vi "AnalogInputVoltageSampleLoop.vi"   [LabVIEW 2018]
uses:
  AnalogInputSample.ctl
  <vilib>/rvi/Emulation/niFpgaGetClockAttributes.vi
  <vilib>/rvi/Emulation/niFpgaSctlEmulationGetInTimedLoop.vi
  <vilib>/rvi/Emulation/niFpgaEmulationReportErrorSimple.vi
  <vilib>/rvi/Emulation/niFpgaEmulationIsFPGAContextNoSignature.vi
  <vilib>/rvi/errors/niFpgaSetErrorForExecOnDevCompSimple.vi
  <vilib>/rvi/eio/common/nirviEmuReportErrorAndStop.vi
  <vilib>/rvi/DataTransferAndStorage/Container/Common/niFpgaContainerGetUniqueNameForEmu.vi
  <vilib>/rvi/FIFO/Fifo_Resource/nirvififoEmulationSetSize.vi
  <vilib>/rvi/FIFO/Fifo_Resource/nirviFifoEmulationQueueMgr.vi
  <instcachedir>/0/nirviFifoEmulationQueueMgr_E5CAEC123FF24DC58D834DCA3CDAA9B5.lvgen/nirviFifoEmulationQueueMgr_E5CAEC123FF24DC58D834DCA3CDAA9B5_002.vi
  <vilib>/Utility/error.llb/Clear Errors.vi
  <vilib>/rvi/FIFO/Fifo_Resource/nirvififoEmulationCreateLock.vi
  <vilib>/rvi/Emulation/niFpgaProcessEmulError.vi
  <vilib>/rvi/FIFO/Fifo_Resource/nirvififoEmulationObtainLock.vi
  <vilib>/rvi/FIFO/Fifo_Resource/nirvififoEmulationReleaseLock.vi
  <vilib>/rvi/occurrence/nirviWaitOnOccurrenceBase.vi
  <vilib>/rvi/errors/nirviReportUnexpectedCaseInternalError.vi
  <vilib>/rvi/errors/nirviReportUnexpectedCaseInternalError (U32).vi
  <vilib>/rvi/eio/common/nirviEmuTemplateMethod_errors.vi
  <vilib>/rvi/Memory/Memory_Emulation/niFpgaMemoryEmulationCacheClearOnFirstRun.vi
  <vilib>/rvi/Memory/Memory_Emulation/nirvimemoryEmulationManagerCache_MakeExclusive.vi
  <vilib>/rvi/Memory/Memory_Emulation/niFpgaMemoryEmulationValidateCache.vi
  <vilib>/rvi/Memory/Memory_Emulation/nirvimemoryEmulationManagerCache_InsertValue.vi
  <vilib>/rvi/Memory/Memory_Emulation/nirvimemoryEmulationManagerCache_ReleaseExclusive.vi
  <vilib>/rvi/Memory/Memory_Emulation/nirvimemoryEmulationManagerCache_GetValue.vi
  <vilib>/rvi/Memory/Memory_Emulation/nirvimemoryEmulationManagerCache_SetValue.vi
  <instcachedir>/0/nirviFifoEmulationQueueMgr_E5CAEC123FF24DC58D834DCA3CDAA9B5.lvgen/nirviFifoEmulationQueueMgr_E5CAEC123FF24DC58D834DCA3CDAA9B5_025.vi
  <vilib>/rvi/FIFO/Fifo_Resource/nirvififoEmulationDetermineInputValidOut.vi
  <vilib>/rvi/Emulation/niFpgaCriticalErrorInLSC.vi
  <vilib>/rvi/DataTransferAndStorage/Container/XNode/niFpgaContainer.xnode
  <vilib>/rvi/FIFO/Fifo_Resource/nirvififoEmulationRead.vi
  <vilib>/eio/EIONode/EIONode.xnode
  <vilib>/rvi/DataTransferAndStorage/Register/Emulation/niFpgaRegisterEmulation.vi
  <vilib>/rvi/FIFO/Fifo_Resource/nirvififoEmulationWrite.vi
types:
  T1 = typedef "AnalogInputSample.ctl" = cluster{"Sample":u64, "Timestamp":u64, "Raw1":sgl, "Raw2":sgl, "Raw3":sgl, "Raw4":sgl, "Raw5":sgl, "Raw6":sgl, "Raw7":sgl, "Raw8":sgl, "Raw9":sgl, "Raw10":sgl, "Raw11":sgl, "Raw12":sgl, "Raw13":sgl, "Raw14":sgl, "Raw15":sgl, "Raw16":sgl}
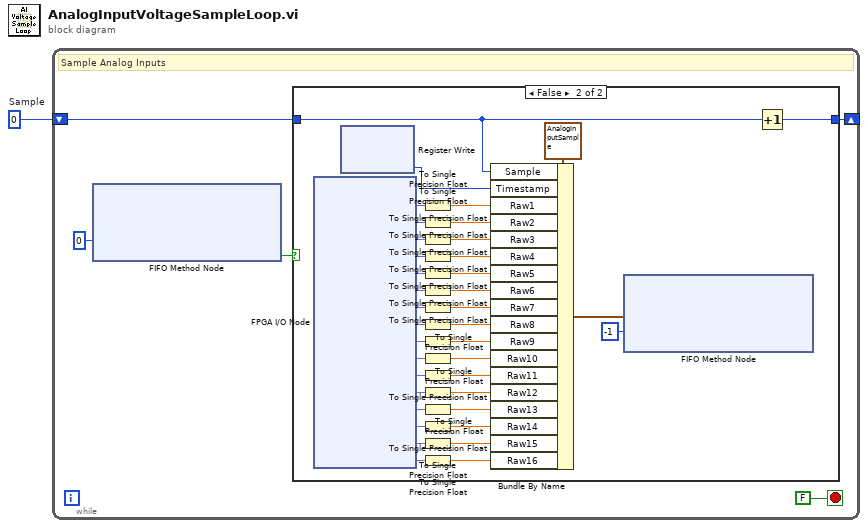
[diagram p0: block diagram]
diagram:
  w1 = u64 0  # Sample
  n1 = while {
    shift-right: [w2] -> _
    shift-left: w1 -> [w3]
    stop <- FALSE stop-if-true
    # "Sample Analog Inputs"
    n2 = xnode ("FIFO Method Node")("Timeout"=0) -> ("Timed Out?"=w5:bool)  [unwired: 1 in, 2 out]
    n3 = case shown="False" w5 {
      tunnel: w3 -> [w7 w27]
      tunnel: [w7 w26] -> w2
      frame True {
      }
      frame False {
        n4 = xnode "FPGA I/O Node"() -> ("Mod1/AI0"=w45:fxp<+/-,24,5>, "Mod1/AI1"=w44:fxp<+/-,24,5>, "Mod1/AI2"=w43:fxp<+/-,24,5>, "Mod1/AI3"=w42:fxp<+/-,24,5>, "Mod1/AI4"=w41:fxp<+/-,24,5>, "Mod1/AI5"=w40:fxp<+/-,24,5>, "Mod1/AI6"=w39:fxp<+/-,24,5>, "Mod1/AI7"=w38:fxp<+/-,24,5>, "Mod1/AI8"=w16:fxp<+/-,24,-4>, "Mod1/AI9"=w17:fxp<+/-,24,-4>, "Mod1/AI10"=w18:fxp<+/-,24,-4>, "Mod1/AI11"=w19:fxp<+/-,24,-4>, "Mod1/AI12"=w20:fxp<+/-,24,-4>, "Mod1/AI13"=w21:fxp<+/-,24,-4>, "Mod1/AI14"=w22:fxp<+/-,24,-4>, "Mod1/AI15"=w23:fxp<+/-,24,-4>)  [unwired: 16 in, 16 out]
        n5 = xnode "Register Write"() -> ("Data"=w25:u64)  [unwired: 1 in, 1 out]
        n6 = To Single Precision Float(number=w45) -> (single precision float=w37:sgl)
        n7 = To Single Precision Float(number=w44) -> (single precision float=w36:sgl)
        n8 = To Single Precision Float(number=w43) -> (single precision float=w35:sgl)
        n9 = To Single Precision Float(number=w42) -> (single precision float=w34:sgl)
        n10 = To Single Precision Float(number=w41) -> (single precision float=w33:sgl)
        n11 = To Single Precision Float(number=w40) -> (single precision float=w32:sgl)
        n12 = To Single Precision Float(number=w39) -> (single precision float=w31:sgl)
        n13 = To Single Precision Float(number=w38) -> (single precision float=w24:sgl)
        n14 = To Single Precision Float(number=w16) -> (single precision float=w15:sgl)
        n15 = To Single Precision Float(number=w17) -> (single precision float=w14:sgl)
        n16 = To Single Precision Float(number=w18) -> (single precision float=w13:sgl)
        n17 = To Single Precision Float(number=w19) -> (single precision float=w12:sgl)
        n18 = To Single Precision Float(number=w20) -> (single precision float=w11:sgl)
        n19 = To Single Precision Float(number=w21) -> (single precision float=w10:sgl)
        n20 = To Single Precision Float(number=w22) -> (single precision float=w9:sgl)
        n21 = To Single Precision Float(number=w23) -> (single precision float=w8:sgl)
        n22 = Bundle By Name(cluster=T1 {"Sample"=0, "Timestamp"=0, "Raw1"=0.0, "Raw2"=0.0, "Raw3"=0.0, "Raw4"=0.0, "Raw5"=0.0, "Raw6"=0.0, "Raw7"=0.0, "Raw8"=0.0, "Raw9"=0.0, "Raw10"=0.0, "Raw11"=0.0, "Raw12"=0.0, "Raw13"=0.0, "Raw14"=0.0, "Raw15"=0.0, "Raw16"=0.0} ("AccelerometerSample"), "Sample"=w27, "Timestamp"=w25, "Raw1"=w37, "Raw2"=w36, "Raw3"=w35, "Raw4"=w34, "Raw5"=w33, "Raw6"=w32, "Raw7"=w31, "Raw8"=w24, "Raw9"=w15, "Raw10"=w14, "Raw11"=w13, "Raw12"=w12, "Raw13"=w11, "Raw14"=w10, "Raw15"=w9, "Raw16"=w8) -> (w30:T1)
        n23 = xnode ("FIFO Method Node")("Element"=w30, "Timeout"=-1) -> ()  [unwired: 1 in, 2 out]
        n24 = Increment(x=w27) -> (x+1=w26:u64)
      }
    }
  }
